vi "PressButton.vi"(8 "ErrorIn":errorcluster caption="Error In", 9 "Button":string, 11 "ObjectIn":refnum<class "ButtonCollection.lvclass"> caption="Object In") -> (0 "ErrorOut":errorcluster caption="Error Out", 1 "SelectedButton":T1, 2 "Valid":bool, 3 "ObjectOut":refnum<class "ButtonCollection.lvclass"> caption="Object Out")   [LabVIEW 2021, in "ButtonCollection.lvclass"]
uses:
  ButtonCollection.lvclass
  ButtonDefinition.ctl
  ButtonCollection.lvclass/ButtonCollection.ctl
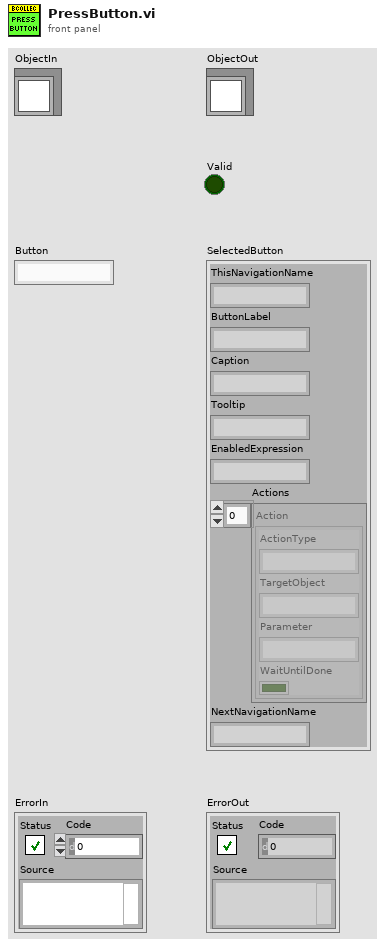
[diagram p1: front panel]
types:
  T1 = typedef "ButtonCollection.lvclass/ButtonDefinition.ctl" = cluster{"ThisNavigationName":string, "ButtonLabel":string, "Caption":string, "Tooltip":string, "EnabledExpression":string, "Actions":cluster{"ActionType":string, "TargetObject":string, "Parameter":string, "WaitUntilDone":bool}[], "NextNavigationName":string}
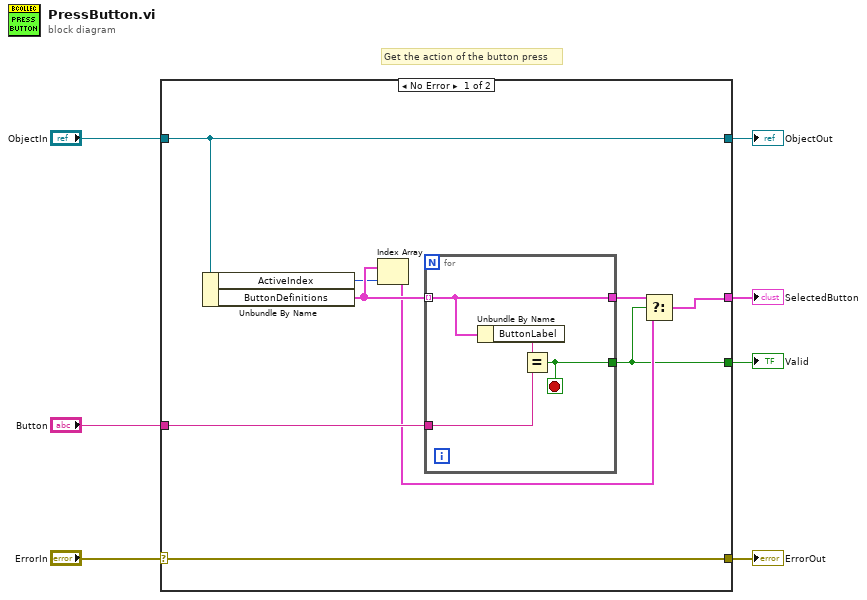
[diagram p0: block diagram]
diagram:
  # "Get the action of the button press"
  n1 = case shown="No Error" "ErrorIn" {
    selector: "ErrorIn" -> [w16 w22]
    tunnel: [w16 w22] -> w6
    tunnel: [w15 w21] -> w4
    tunnel: "ObjectIn" -> [w15 w21]
    tunnel: "Button" -> [w14 _]
    tunnel: [w10 _] -> w2
    tunnel: [w8 _] -> w1
    frame No Error {
      n2 = Unbundle By Name(w15) -> ("ActiveIndex"=w12:i32, "ButtonDefinitions"=w13:T1[])
      n3 = Index Array(array=w13, index=w12) -> (element=w11:T1)
      n4 = for {
        tunnel: w13 -> [w18] mode=indexing
        tunnel: w14 -> [w19]
        tunnel: [w18] -> w9
        tunnel: [w17] -> w8
        stop <- w17 stop-if-true
        n5 = Unbundle By Name(w18) -> ("ButtonLabel"=w20:string)
        n6 = Equal?(x=w20, y=w19) -> (x = y?=w17:bool)
      }
      n7 = Select(t=w9, s=w8, f=w11) -> (s? t:f=w10:T1)
    }
    frame Error {
    }
  }
  "ErrorOut" <- w6
  "ObjectOut" <- w4
  "SelectedButton" <- w2
  "Valid" <- w1
